vi "setAxisObject.vi"(8 "error in (no error)":errorcluster, 9 "Axis Object":refnum<class "Axis.lvclass">, 10 "Axis Letter":string, 11 "Controller in":refnum<class "Controller.lvclass">) -> (0 "error out":errorcluster, 3 "Controller out":refnum<class "Controller.lvclass">)   [LabVIEW 2019, in "Controller.lvclass"]
uses:
  Controller.lvclass
  Axis/Axis.lvclass
  Controller.lvclass/Controller.ctl
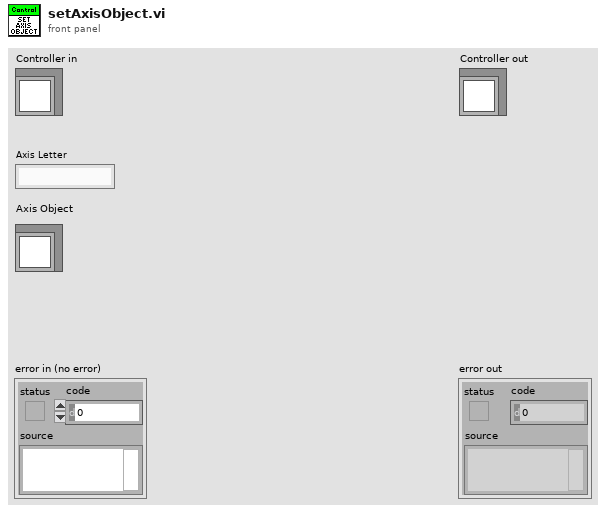
[diagram p1: front panel]
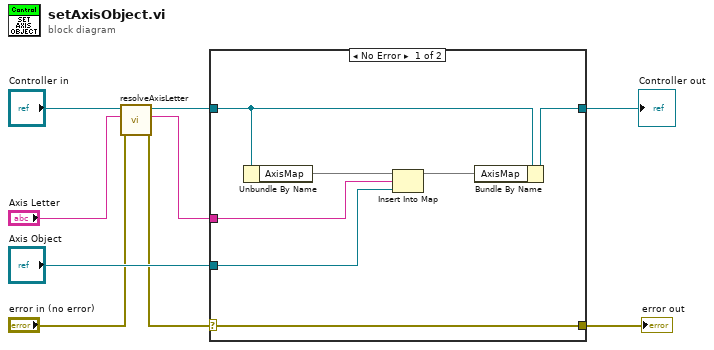
[diagram p0: block diagram]
diagram:
  n1 = call "resolveAxisLetter.vi"("error in (no error)"="error in (no error)", "Axis Letter in"="Axis Letter", "Controller in"="Controller in") -> ("error out"=w5:errorcluster, "Axis Letter out"=w1:string, "Controller out"=w3:refnum<class "Controller.lvclass">)  [unwired: 6 in]
  n2 = case shown="No Error" w5 {
    selector: w5 -> [w16 w18]
    tunnel: [w16 w18] -> w9
    tunnel: [w14 w17] -> w8
    tunnel: w3 -> [w13 w17]
    tunnel: w1 -> [w10 _]
    tunnel: "Axis Object" -> [w11 _]
    frame No Error {
      n3 = Unbundle By Name(w13) -> ("AxisMap"=w15:map{string, refnum<class "Axis.lvclass">})
      n4 = Insert Into Map(map in=w15, key=w10, value=w11) -> (map out=w12:map{string, refnum<class "Axis.lvclass">})  [unwired: 2 out]
      n5 = Bundle By Name(cluster=w13, "AxisMap"=w12) -> (w14:refnum<class "Controller.lvclass">)
    }
    frame Error {
    }
  }
  "error out" <- w9
  "Controller out" <- w8
